vi "VI Fehlerliste.vi"() -> ()   [LabVIEW 2020, in "cRIO Ueberwachung.lvlib"]
uses:
  cRIO Ueberwachung.lvlib
  Visualisierungs Elemente/Button.ctl
  Sprachverwaltung/FGV Aktion Tabelle zerlegen.ctl
  FGV Fehlerliste Aktionen.ctl
  Allgemein/allgemeine Sub-VIs.lvlib
  Sprachverwaltung/Sprachverwaltung.lvlib
panel:
  in  "Quittieren":T1
  out "Tabelle Puffer":string[][](table)
  out "Tabelle Aktuell":string[][](table)
  in  "Stopp":T1
  # "Fehler Steuerung"
  # "Aktuelle Fehler"
  # "Fehler Puffer"
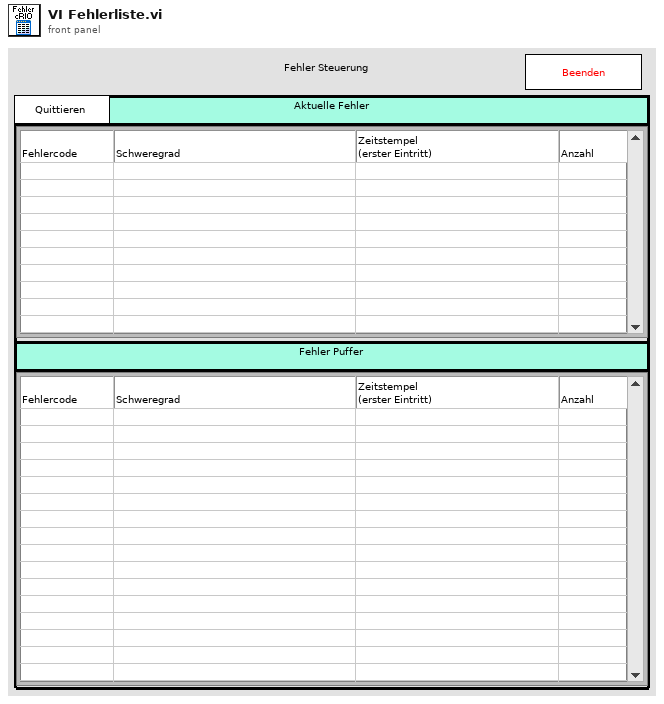
[diagram p1: front panel]
types:
  T1 = typedef "Button.ctl" = bool
  T2 = typedef "Sprachverwaltung.lvlib/FGV Aktion Tabelle zerlegen.ctl" = enum16{"laden", "vereinzeln", "speichern"}
  T3 = typedef "cRIO Ueberwachung.lvlib/FGV Fehlerliste Aktionen.ctl" = enum16{"lesen", "abfragen", "löschen", "laden", "speichern"}
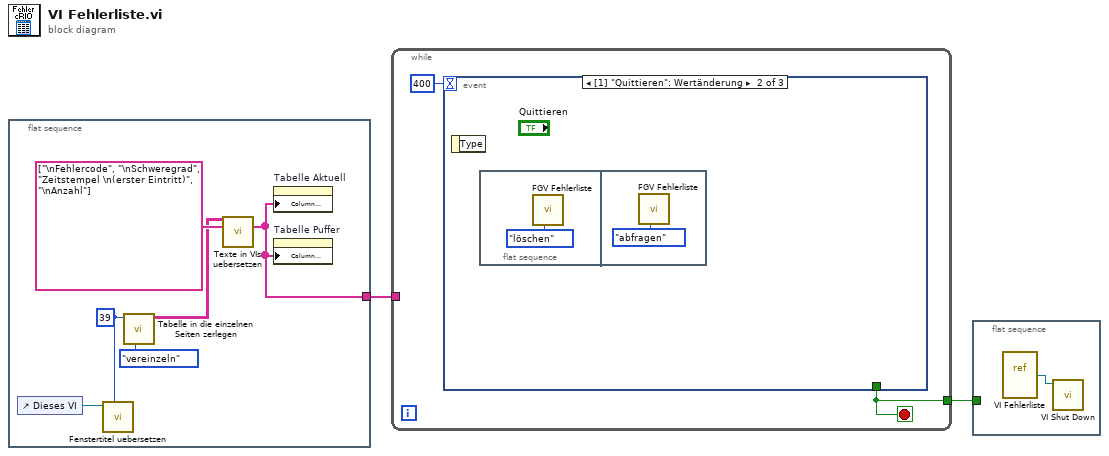
[diagram p0: block diagram]
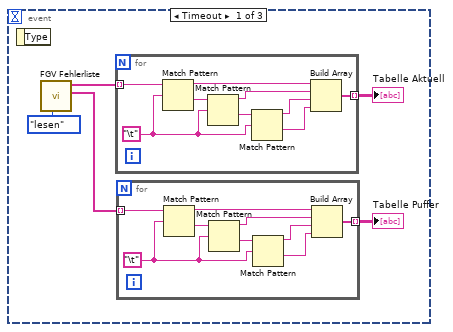
[diagram p2: hidden frame]
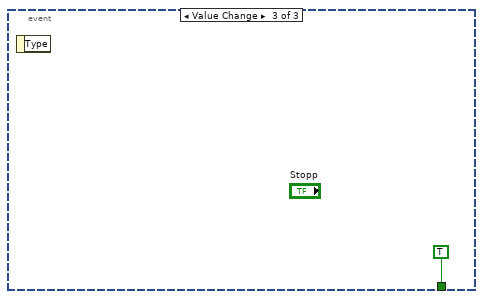
[diagram p3: hidden frame]
diagram:
  n1 = flat-sequence {
    tunnel: [w7] -> w2
    frame #0 {
      w4 = 39 ("Index (Seite)")
      n2 = control-ref of="Dieses VI"() -> (w5:refnum<vi>)
      n3 = call "Fenstertitel uebersetzen.vi"("Index (Seite)"=w4, "Dieses VI"=w5) -> ()  [unwired: 6 in, 4 out]
      n4 = call "Tabelle in die einzelnen Seiten zerlegen.vi"("Aktion"=FGV_Aktion_Tabelle_zerlegen."vereinzeln", "Index (Seite)"=w4) -> ("Sprachliste"=w6:string[][])  [unwired: 7 in, 2 out]
      n5 = call "Texte in VIs uebersetzen.vi"("Sprachliste"=w6, "String-Array zum Übersetzen"=string[] ["\nFehlercode", "\nSchweregrad", "Zeitstempel \n(erster Eintritt)", "\nAnzahl"] ("Spaltentitel[]")) -> ("String-Array zum Übersetzen"=w7:string[])  [unwired: 9 in, 4 out]
      n6 = property on="Tabelle Aktuell" class="Tbl (strikt)"("Column Headers[]"=w7) -> ()  [unwired: 2 in, 2 out]
      n7 = property on="Tabelle Puffer" class="Tbl (strikt)"("Column Headers[]"=w7) -> ()  [unwired: 2 in, 2 out]
    }
  }
  n8 = while {
    tunnel: w2 -> [_]
    tunnel: [w9] -> w1
    stop <- w9 stop-if-true
    n9 = event shown="[1] \"Quittieren\": Wertänderung" {
      selector: _ -> [_ _ _]
      dyn-events: _ -> [_ _ _]
      timeout: 400 -> [_ _ _]
      tunnel: [_ _ TRUE] -> w9
      event Timeout {
        n10 = event-data() -> ()  [unwired: 1 in, 1 out]
        n11 = call "FGV Fehlerliste.vi"("Aktionen Fehlerliste"=FGV_Fehlerliste_Aktionen."lesen") -> ("Gespeicherte Fehler"=w15:string[], "Aktuelle Fehler"=w14:string[])  [unwired: 9 in]
        n12 = for {
          tunnel: w14 -> [w33] mode=indexing
          tunnel: [w25] -> w12 mode=indexing
          w30 = "\t"
          n13 = Match Pattern(string=w33, regular expression=w30) -> (before substring=w29:string, after substring=w32:string)  [unwired: 1 in, 2 out]
          n14 = Match Pattern(string=w32, regular expression=w30) -> (before substring=w28:string, after substring=w31:string)  [unwired: 1 in, 2 out]
          n15 = Match Pattern(string=w31, regular expression=w30) -> (before substring=w27:string, after substring=w26:string)  [unwired: 1 in, 2 out]
          n16 = Build Array(w29, w28, w27, w26) -> (w25:string[])
        }
        "Tabelle Aktuell" <- w12
        n17 = for {
          tunnel: w15 -> [w24] mode=indexing
          tunnel: [w16] -> w11 mode=indexing
          w21 = "\t"
          n18 = Match Pattern(string=w24, regular expression=w21) -> (before substring=w20:string, after substring=w23:string)  [unwired: 1 in, 2 out]
          n19 = Match Pattern(string=w23, regular expression=w21) -> (before substring=w19:string, after substring=w22:string)  [unwired: 1 in, 2 out]
          n20 = Match Pattern(string=w22, regular expression=w21) -> (before substring=w18:string, after substring=w17:string)  [unwired: 1 in, 2 out]
          n21 = Build Array(w20, w19, w18, w17) -> (w16:string[])
        }
        "Tabelle Puffer" <- w11
      }
      event Value Change {
        n22 = event-data() -> ()  [unwired: 1 in, 1 out]
        n23 = flat-sequence {
          frame #0 {
            n24 = call "FGV Fehlerliste.vi"("Aktionen Fehlerliste"=FGV_Fehlerliste_Aktionen."löschen") -> ()  [unwired: 9 in, 2 out]
          }
          frame #1 {
            n25 = call "FGV Fehlerliste.vi"("Aktionen Fehlerliste"=FGV_Fehlerliste_Aktionen."abfragen") -> ()  [unwired: 9 in, 2 out]
          }
        }
      }
      event Value Change {
        n26 = event-data() -> ()  [unwired: 1 in, 1 out]
      }
    }
  }
  n27 = flat-sequence {
    tunnel: w1 -> [_]
    frame #0 {
      n28 = vi-ref "VI Fehlerliste.vi"() -> (w37:refnum<vi>)
      n29 = call "VI Shut Down.vi"("VI Referenz"=w37) -> ()  [unwired: 11 in]
    }
  }
